vi "Read_Joint_Data.vi"(11 "CAN Frame":T2 {"payload" format="%x"; "timestamp" format="%<%I:%M:%S%8u %p\n%x>T"; "identifier" format="%x"}) -> (2 "Actual position":u16, 3 "Joint Position out":T3)   [LabVIEW 2015]
uses:
  <vilib>/Stratom, Inc/X-CAN for myRIO (API)/X-CAN Class/Type Definitions/CANFrame.ctl
  <vilib>/Stratom, Inc/X-CAN for myRIO (API)/X-CAN Class/X-CAN.lvclass
panel:
  in  "Joint Position in":T1
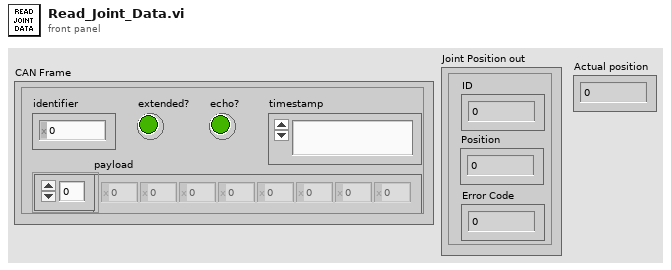
[diagram p1: front panel]
types:
  T1 = cluster{"ID":u8, "Position":u16, "Error Code":u8}
  T2 = typedef "X-CAN.lvclass/CANFrame.ctl" = cluster{"identifier":u32, "extended?":bool, "echo?":bool, "payload":u8[], "timestamp":timestamp}
  T3 = cluster{"Error Code":u8, "Position":u16, "ID":u8}
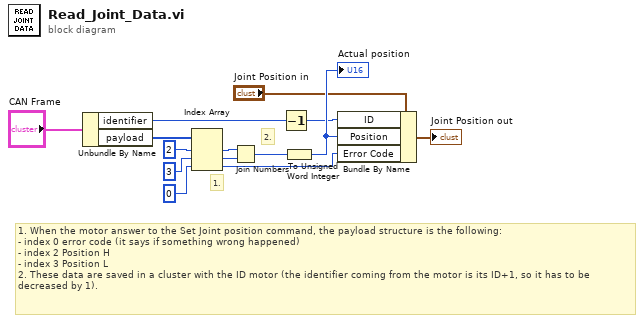
[diagram p0: block diagram]
diagram:
  # "2."
  # "1."
  # "1. When the motor answer to the Set Joint position command, the payload structure is the following:\n- index 0 error code (it says if something wrong happened)\n- index 2 Position H\n- index 3 Position L\n2. These data are saved in a cluster with the ID motor (the identifier coming from the motor is its ID+1, so it has to be \ndecreased by 1)."
  n1 = Unbundle By Name("CAN Frame") -> ("identifier"=w3:u32, "payload"=w4:u8[])
  n2 = Index Array(array=w4, index #1=2 ("index"), index #2=3 ("index"), index #3=0 ("index")) -> (element #1=w7:u8, element #2=w8:u8, element #3=w13:u8)
  n3 = Join Numbers(hi=w7, lo=w8) -> ((hi.lo)=w11:u16)
  n4 = Decrement(x=w3) -> (x-1=w9:u32)
  n5 = To Unsigned Word Integer(number=w11) -> (unsigned 16bit integer=w12:u16)
  "Actual position" <- w12
  n6 = Bundle By Name(cluster="Joint Position in", "ID"=w9, "Position"=w12, "Error Code"=w13) -> (→"Joint Position out":T1)
